vi "Initialize.vi"(8 "error in (no error)":errorcluster, 9 "Reset (True)":bool=TRUE, 10 "ID Query (True)":bool=TRUE, 11 "VISA resource name":refnum<visa-resource-name>) -> (0 "error out":errorcluster, 3 "VISA resource name out":refnum<visa-resource-name>)   [LabVIEW 2014, in "FG Simulator.lvlib"]
doc: "Establishes communication with the instrument and optionally performs an instrument identification query and/or an instrument reset. It also places the instrument in a default state needed for other instrument driver operations. Therefore, call this VI before calling other instrument driver VIs for this instrument. Generally, you need to call the Initialize VI only once at the beginning of an application."
uses:
  FG Simulator.lvlib
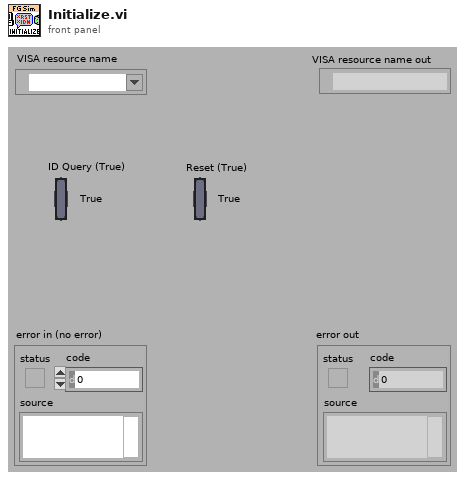
[diagram p1: front panel]
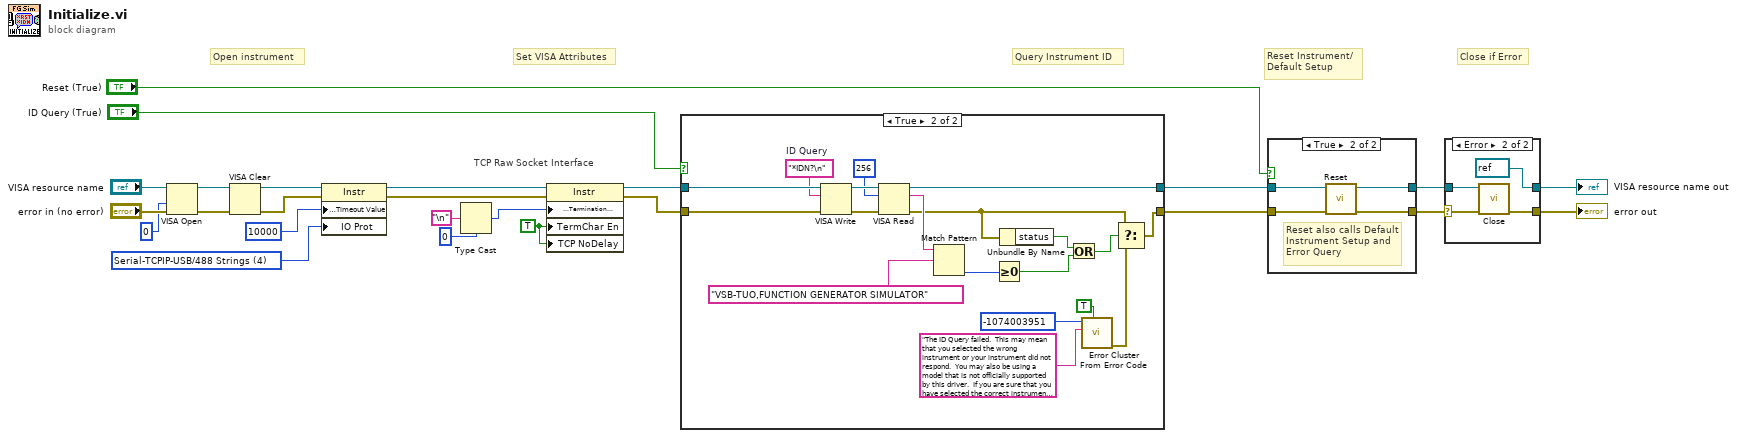
[diagram p0: block diagram]
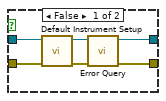
[diagram p4: hidden frame]
diagram:
  w8 = TRUE ("Message Based Settings:Termination Character Enable")
  w12 = u16 4 items=["Normal"=1, "VXI/FDC"=2, "GPIB/HS488"=3, "Serial-TCPIP-USB/488 Strings"=4, "USBTMC/Vendor-Specific"=5] ("Message Based Settings:IO Protocol")
  # "TCP Raw Socket Interface"
  # "Set VISA Attributes"
  # "Close if Error"
  # "Query Instrument ID"
  # "Reset Instrument/\nDefault Setup"
  # "Open instrument"
  n1 = VISA Open(access mode=u32 0, error in (no error)="error in (no error)", VISA resource name="VISA resource name") -> (VISA resource name=w20:refnum<visa-resource-name>, error out=w19:errorcluster)  [unwired: 2 in]
  n2 = VISA Clear(VISA resource name=w20, error in (no error)=w19) -> (VISA resource name out=w18:refnum<visa-resource-name>, error out=w17:errorcluster)
  n3 = property class="Instr"(reference=w18, error in=w17, "General Settings:Timeout Value"=u32 10000, "IO Prot"=w12) -> (reference out=w7:refnum<visa-resource-name>, error out=w6:errorcluster)
  n4 = Type Cast(type=u8 0, x="\n" ("Line Feed Constant")) -> (*(type *) &x=w9:u8)
  n5 = property class="Instr"(reference=w7, error in=w6, "Message Based Settings:Termination Character"=w9, "TermChar En"=w8, "TCP NoDelay"=w8) -> (reference out=w4:refnum<visa-resource-name>, error out=w1:errorcluster)
  n6 = case shown="True" "ID Query (True)" {
    tunnel: [w26 w46] -> w3
    tunnel: [w27 w43] -> w2
    tunnel: w4 -> [w27 w44]
    tunnel: w1 -> [w26 w45]
    frame False {
    }
    frame True {
      w37 = "*IDN?\n"  # ID Query
      n7 = VISA Write(VISA resource name=w44, write buffer=w37, error in (no error)=w45) -> (VISA resource name out=w41:refnum<visa-resource-name>, error out=w40:errorcluster)  [unwired: 1 out]
      n8 = VISA Read(VISA resource name=w41, byte count=u32 256, error in (no error)=w40) -> (VISA resource name out=w43:refnum<visa-resource-name>, read buffer=w42:string, error out=w31:errorcluster)  [unwired: 1 out]
      n9 = Match Pattern(string=w42, regular expression="VSB-TUO,FUNCTION GENERATOR SIMULATOR") -> (offset past match=w32:i32)  [unwired: 1 in, 3 out]
      n10 = Greater Or Equal To 0?(x=w32) -> (x >= 0?=w29:bool)
      n11 = Unbundle By Name(w31) -> ("status"=w30:bool)
      n12 = Or(x=w30, y=w29) -> (x .or. y?=w28:bool)
      n13 = call <vilib>:"Error Cluster From Error Code.vi"("show call chain? (False)"=TRUE, "error message (\"\")"="The ID Query failed.  This may mean that you selected the wrong instrument or your instrument did not respond.  You may also be using a model that is not officially supported by this driver.  If you are sure that you have selected the correct instrument and it is responding, try disabling the ID Query." ("Source (VI Name)"), "error code (0)"=-1074003951 ("Code")) -> ("error out"=w36:errorcluster)  [unwired: 6 in]
      n14 = Select(t=w31, s=w28, f=w36) -> (s? t:f=w46:errorcluster)
    }
  }
  n15 = case shown="True" "Reset (True)" {
    tunnel: w3 -> [w51 w53]
    tunnel: [w48 w56] -> w13
    tunnel: w2 -> [w52 w54]
    tunnel: [w49 w55] -> w14
    frame False {
      n16 = call "Default Instrument Setup.vi"("error in (no error)"=w51, "VISA resource name"=w52) -> ("error out"=w47:errorcluster, "VISA resource name out"=w50:refnum<visa-resource-name>)  [unwired: 8 in]
      n17 = call "Error Query.vi"("error in (no error)"=w47, "VISA resource name"=w50) -> ("error out"=w48:errorcluster, "VISA resource name out"=w49:refnum<visa-resource-name>)  [unwired: 6 in, 2 out]
    }
    frame True {
      # "Reset also calls Default Instrument Setup and Error Query"
      n18 = call "Reset.vi"("error in (no error)"=w53, "VISA resource name"=w54) -> ("error out"=w56:errorcluster, "VISA resource name out"=w55:refnum<visa-resource-name>)  [unwired: 8 in]
    }
  }
  n19 = case shown="Error" w13 {
    selector: w13 -> [w57 w60]
    tunnel: w14 -> [w58 w61]
    tunnel: [w58 refnum<visa-resource-name> refnum ("VISA resource name out")] -> w16
    tunnel: [w57 w62] -> w15
    frame No Error {
    }
    frame Error {
      n20 = call "Close.vi"("error in (no error)"=w60, "VISA resource name"=w61) -> ("error out"=w62:errorcluster)  [unwired: 9 in]
    }
  }
  "VISA resource name out" <- w16
  "error out" <- w15
